vi "TOF TOGGLE.vi"(9 "Delay (ms)":u32=500, 10 "Input":bool) -> (2 "Output":bool)   [LabVIEW 2016]
doc: "Similar to a toggle, with a TOF timer built in.\nThe TOF TOGGLE, when given a True input, will immediately output true. When the input reverts back to False, the output will wait for the specified delay to elapse before outputting False.\n\nIf the Delay is set to 0, this will simply act as a toggle."
panel:
  in  "Delay_TOF":T1
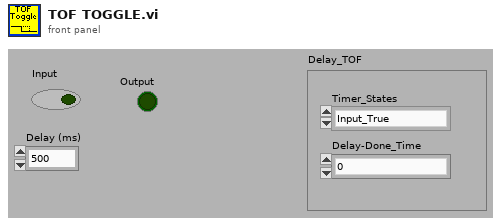
[diagram p1: front panel]
types:
  T1 = cluster{"Timer_States":enum16{"Input_True", "Input_False_Timing", "Input_False_Timing_Complete"}, "Delay-Done_Time":u32}
  T2 = enum16{"Input_True", "Input_False_Timing", "Input_False_Timing_Complete"}
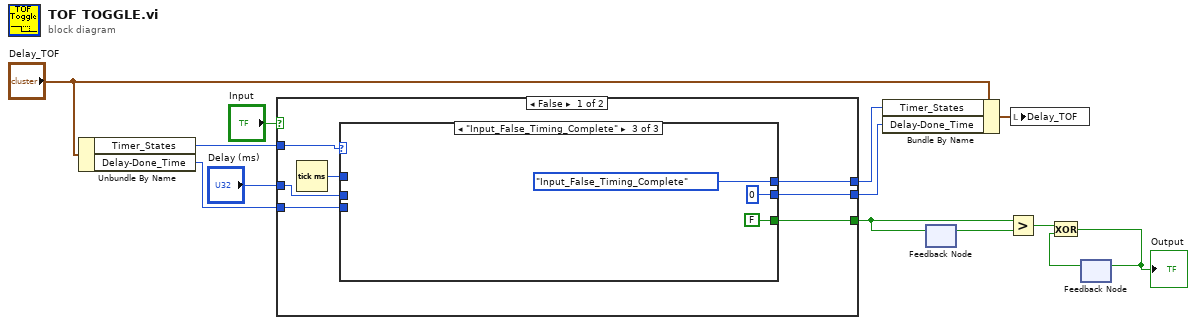
[diagram p0: block diagram]
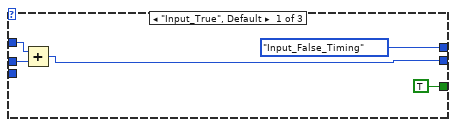
[diagram p2: hidden frame]
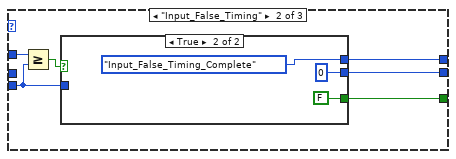
[diagram p3: hidden frame]
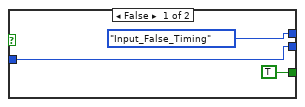
[diagram p4: hidden frame]
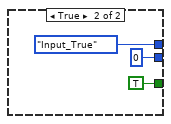
[diagram p5: hidden frame]
diagram:
  n1 = Unbundle By Name("Delay_TOF") -> ("Timer_States"=w10:T2, "Delay-Done_Time"=w8:u32)
  n2 = case shown="False" "Input" {
    tunnel: [w17 TRUE] -> w2
    tunnel: [w18 T2."Input_True" ("Timer_States")] -> w6
    tunnel: [w19 u32 0 ("Delay-Done_Time")] -> w7
    tunnel: w10 -> [w16 _]
    tunnel: "Delay (ms)" -> [w15 _]
    tunnel: w8 -> [w14 _]
    frame False {
      n3 = Tick Count (ms)() -> (millisecond timer value=w20:u32)
      n4 = case shown="\"Input_False_Timing_Complete\"" w16 {
        tunnel: w20 -> [w24 w31 _]
        tunnel: [w23 w27 u32 0 ("Delay-Done_Time")] -> w19
        tunnel: [T2."Input_False_Timing" ("Timer_States") w29 T2."Input_False_Timing_Complete" ("Timer_States")] -> w18
        tunnel: [TRUE w28 FALSE] -> w17
        tunnel: w15 -> [w21 _ _]
        tunnel: w14 -> [_ w26 _]
        frame "Input_True", Default {
          n5 = Add(x=w24, y=w21) -> (x+y=w23:u32)
        }
        frame "Input_False_Timing" {
          n6 = Greater Or Equal?(x=w31, y=w26) -> (x >= y?=w30:bool)
          n7 = case shown="True" w30 {
            tunnel: [T2."Input_False_Timing" ("Timer_States") T2."Input_False_Timing_Complete" ("Timer_States")] -> w29
            tunnel: [TRUE FALSE] -> w28
            tunnel: [w32 u32 0 ("Delay-Done_Time")] -> w27
            tunnel: w26 -> [w32 _]
            frame False {
            }
            frame True {
            }
          }
        }
        frame "Input_False_Timing_Complete" {
        }
      }
    }
    frame True {
    }
  }
  n8 = Bundle By Name(cluster="Delay_TOF", "Timer_States"=w6, "Delay-Done_Time"=w7) -> (w12:T1)
  n9 = feedback #1() -> (w5:bool)  [unwired: 1 in]
  n10 = feedback-in #1(w2) -> ()
  n11 = Greater?(x=w2, y=w5) -> (0:w4:bool)
  n12 = local write "Delay_TOF"(w12) -> ()
  n13 = feedback #2() -> (w3:bool)  [unwired: 1 in]
  n14 = Exclusive Or(1:w3, 2:w4) -> (0:w1:bool)
  "Output" <- w1
  n15 = feedback-in #2(w1) -> ()
